vi "setStandardButtons.vi"(8 "Error In":errorcluster, 10 "buttons":T1 items=["NoButton"=0, "Ok"=1024, "Save"=2048, "SaveAll"=4096, "Open"=8192, "Yes"=16384, "YesToAll"=32768, "No"=65536, "NoToAll"=131072, "Abort"=262144, "Retry"=524288, "Ignore"=1048576, "Close"=2097152, "Cancel"=4194304, "Discard"=8388608, "Help"=16777216, "Apply"=33554432, "Reset"=67108864, "RestoreDefaults"=134217728], 11 "QMessageBox In":refnum<class "QMessageBox.lvclass">) -> (0 "Error Out":errorcluster, 3 "QMessageBox Out":refnum<class "QMessageBox.lvclass">)   [LabVIEW 2014, in "QMessageBox.lvclass"]
doc: "LabVIEW-specific documentation is not yet available. See <b>http://doc.qt.io/qt-5/QMessageBox.html#setStandardButtons</b>"
uses:
  QMessageBox.lvclass
  StandardButton.ctl
  LQ Core/LQIdentity/LQIdentity.lvclass/LQIdentity.ctl
  LQ Core/LQ Core.lvlib
  LQ Core/LQIdentity/LQIdentity.lvclass
panel:
  # "Copyright (c) 2016 Sze Howe Koh\n\nThis Source Code Form is subject to the terms of the Mozilla Public\nLicense, v. 2.0. If a copy of the MPL was not distributed with this\nfile, You can obtain one at http://mozilla.org/MPL/2.0/."
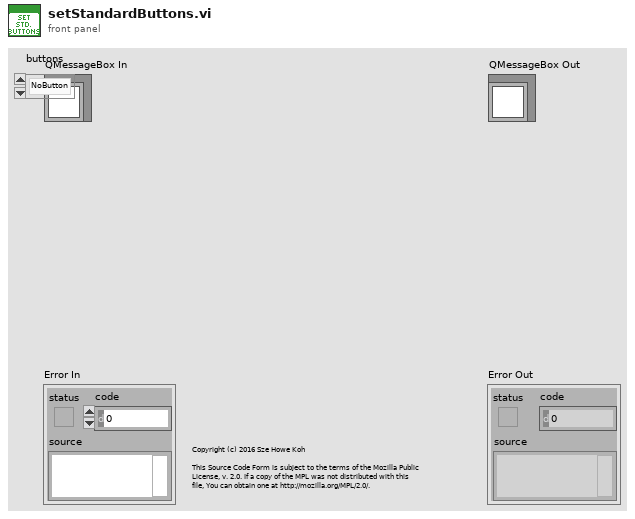
[diagram p1: front panel]
types:
  T1 = typedef "QMessageBox.lvclass/StandardButton.ctl" = i32
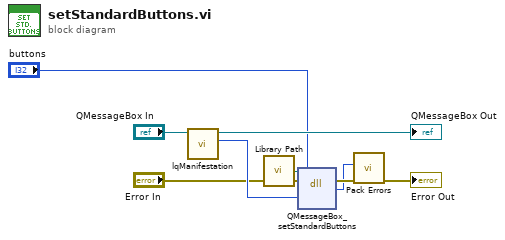
[diagram p0: block diagram]
diagram:
  n1 = call "lqManifestation.vi"("LQIdentity in"="QMessageBox In") -> ("Manifestation"=w6:u64, "LQIdentity out"=→"QMessageBox Out":refnum<class "QMessageBox.lvclass">)  [unwired: 9 in]
  n2 = call "Library Path.vi"() -> ("Library Path"=w7:path)
  n3 = dll-call lib="?" fn="QMessageBox_setStandardButtons"(path in=w7, error in="Error In", "_instance"=w6, "buttons"="buttons") -> (error out=w4:errorcluster, w2:i32)  [unwired: 3 in, 1 out]
  n4 = call "Pack Errors.vi"("Error In"=w4, "Error Code"=w2) -> ("Error Out"=→"Error Out":errorcluster)  [unwired: 9 in]
